vi "sample6(OPMode).vi"() -> ()   [LabVIEW 2011]
uses:
  <vilib>/Platform/TimedLoop/XDataNode/timing_clust.ctl
  <vilib>/Platform/TimedLoop/XDataNode/nitl_modes.ctl
  <vilib>/Platform/TimedLoop/XDataNode/wakeup.ctl
  <vilib>/Platform/TimedLoop/XDataNode/XDataNode.xnode
  <vilib>/Platform/TimedLoop/XDataNode/XDNodeRunTimeDep.lvlib
  user32.dll
panel:
  in  "Mode":u8(slide) scale=0.0..3.0
  out "change mode":bool
  out "Chart":cluster{"MovingSpeed":i16, "Present Speed":i16}(graph)
  out "Present Value":i16
  out "STOP2":bool
  in  "ID":u8=1 max=253
  in  "Baudrate":u32=1000000
  in  "COM":refnum<visa-resource-name> caption="COMポート"
  in  "STOP":bool
  in  "Value":i16(knob) scale=0.0..4095.0
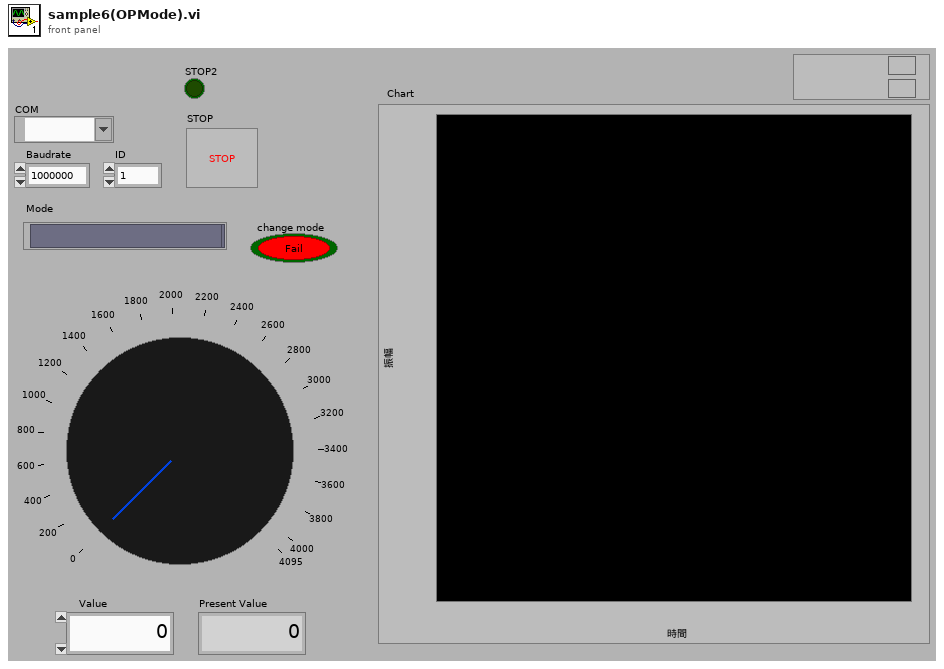
[diagram p1: front panel]
types:
  T1 = typedef "XDNodeRunTimeDep.lvlib/timing_clust.ctl" = cluster{"Expected End [f-1]":u64, "Actual End [f-1]":u64, "Finished Late? [f-1]":bool, "Expected End [i-1]":u64, "Actual End [i-1]":u64, "Finished Late? [i-1]":bool, "Expected Start [i]":u64, "Actual Start [i]":u64, "Expected Start [f]":u64, "Actual Start [f]":u64, "Source Name":string, "Structure Name":string, "Period":i64, "Deadline":i64, "Offset":i64, "Start":i64, "Priority":i32, "Timeout":i32, "Mode":T2, "Wakeup Reason":T3, "Error":errorcluster, "Source Type":string, "Secondary Source Type":string, "Global End Time":u64, "Global Start Time":u64, "Frame Duration":u64, "Iteration Duration":u64, "Assigned CPU":i32, "I/O Scan Engine Mode":u32}
  T2 = typedef "XDNodeRunTimeDep.lvlib/nitl_modes.ctl" = enum32{"No Change", "Process missed periods, maintain original phase", "Discard missed periods, maintain original phase", "Process missed periods, ignore original phase", "Discard missed periods, ignore original phase"}
  T3 = typedef "XDNodeRunTimeDep.lvlib/wakeup.ctl" = enum32{"Normal", "Aborted", "Asynchronous wakeup", "Timing source error", "Timed loop error", "Timeout"}
  T4 = enum16{"Joint", "Wheel", "Multi Turn", "unknown"}
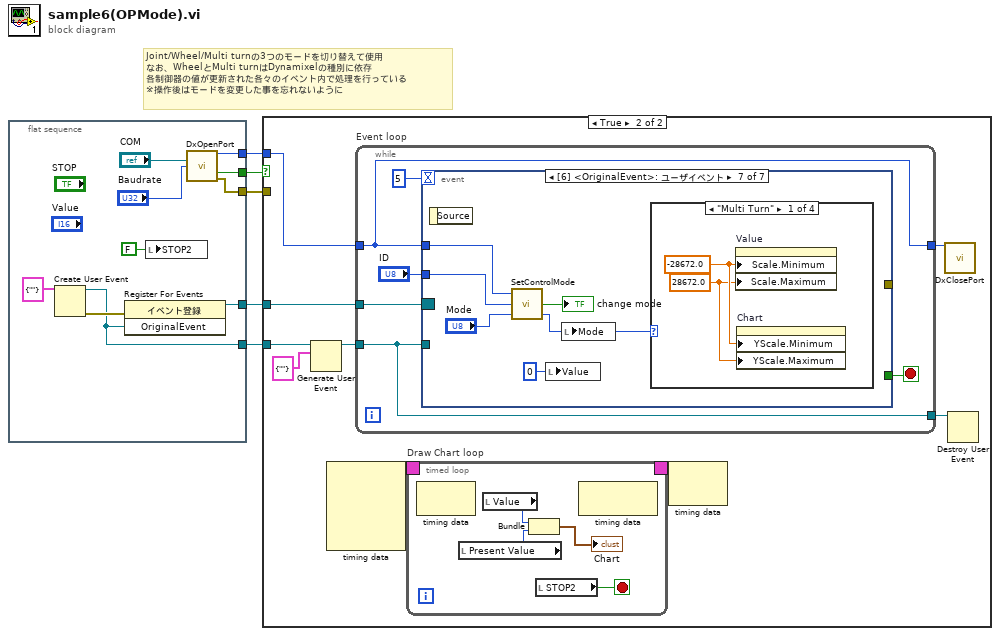
[diagram p0: block diagram]
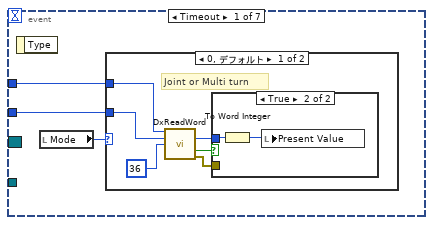
[diagram p3: hidden frame]
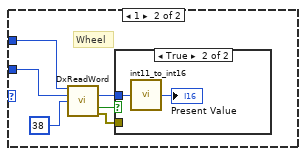
[diagram p5: hidden frame]
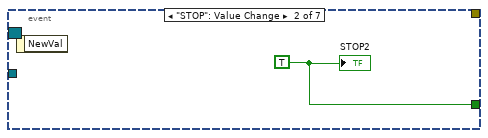
[diagram p7: hidden frame]
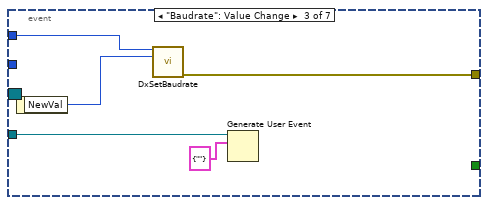
[diagram p8: hidden frame]
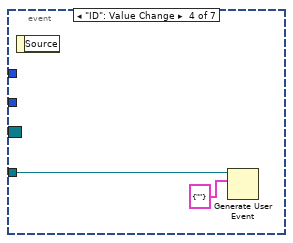
[diagram p9: hidden frame]
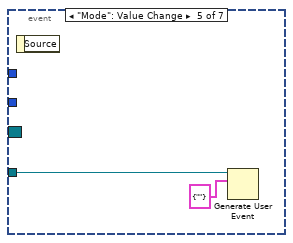
[diagram p10: hidden frame]
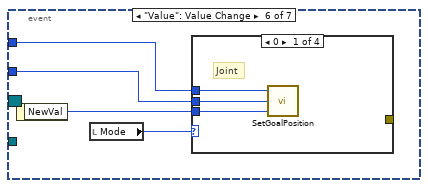
[diagram p11: hidden frame]
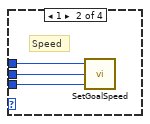
[diagram p12: hidden frame]
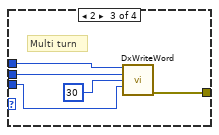
[diagram p13: hidden frame]
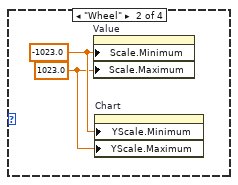
[diagram p15: hidden frame]
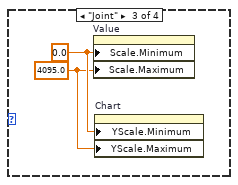
[diagram p16: hidden frame]
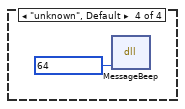
[diagram p17: hidden frame]
diagram:
  # "Joint/Wheel/Multi turnの3つのモードを切り替えて使用\nなお、WheelとMulti turnはDynamixelの種別に依存\n各制御器の値が更新された各々のイベント内で処理を行っている\n※操作後はモードを変更した事を忘れないように"
  n1 = flat-sequence {
    tunnel: [w13] -> w5
    tunnel: [w12] -> w4
    tunnel: [w11] -> w3
    tunnel: [w7] -> w2
    tunnel: [w6] -> w1
    frame #0 {
      n2 = Create User Event(user event datatype=cluster{"string":string} {"string"=""} ("OriginalEvent")) -> (user event=w6:refnum<user-event>, error out=w9:errorcluster)  [unwired: 1 in]
      n3 = register-events(error in=w9, w6) -> (reference out=w7:refnum<event-registration>)  [unwired: 1 in, 1 out]
      n4 = local write "STOP2"(FALSE ("STOP2")) -> ()
      n5 = call "DxOpenPort.vi"("port"="COM", "baudrate"="Baudrate") -> ("dvid"=w13:u32, "成功"=w12:bool, "エラー出力"=w11:errorcluster)  [unwired: 11 in]
    }
  }
  n6 = case shown="TRUE" w4 {
    tunnel: w5 -> [_ w22]
    tunnel: w3 -> [_ _]
    tunnel: w2 -> [_ w20]
    tunnel: w1 -> [_ w18]
    frame False {
    }
    frame True {
      n7 = Generate User Event(user event=w18, event data cluster=cluster{"string":string} {"string"=""} ("イベントデータ")) -> (user event out=w17:refnum<user-event>)  [unwired: 1 in, 1 out]
      n8 = node-c288() -> (w24:T1)  [unwired: 4 in]
      n9 = while "Event loop" {
        tunnel: w22 -> [w25]
        tunnel: [w25] -> w21
        tunnel: w20 -> [w27]
        tunnel: w17 -> [w26]
        tunnel: [w26] -> w16
        stop <- w30 stop-if-true
        n10 = event shown="[6] <OriginalEvent>: ユーザイベント" {
          selector: w27 -> [_ _ _ _ _ _ _]
          dyn-events: _ -> [_ _ _ _ _ _ _]
          timeout: 5 -> [_ _ _ _ _ _ _]
          tunnel: w25 -> [w33 _ w55 _ _ w62 w80]
          tunnel: [_ w50 _ _ _ _ _] -> w30
          tunnel: "ID" -> [w32 _ _ _ _ w60 w75]
          tunnel: w26 -> [_ _ w52 w56 w58 _ _]
          tunnel: [_ _ w51 _ _ _ _] -> _
          event Timeout {
            n11 = event-data() -> ()  [unwired: 1 in, 1 out]
            n12 = local read "Mode"() -> (w31:u8)
            n13 = case shown="0, デフォルト" w31 {
              tunnel: w33 -> [w35 w43]
              tunnel: w32 -> [w34 w42]
              frame 0, Default {
                # "Joint or Multi turn"
                n14 = call "DxReadWord.vi"("dvid in"=w35, "id"=w34, "address"=u16 36) -> ("data out"=w37:u16, "成功"=w38:bool, "エラー出力"=w39:errorcluster)  [unwired: 9 in, 1 out]
                n15 = case shown="TRUE" w38 {
                  tunnel: w37 -> [_ w41]
                  tunnel: w39 -> [_ _]
                  frame False {
                  }
                  frame True {
                    n16 = To Word Integer(number=w41) -> (16bit integer=w40:i16)
                    n17 = local write "Present Value"(w40) -> ()
                  }
                }
              }
              frame 1 {
                # "Wheel"
                n18 = call "DxReadWord.vi"("dvid in"=w43, "id"=w42, "address"=u16 38) -> ("data out"=w45:u16, "成功"=w46:bool, "エラー出力"=w47:errorcluster)  [unwired: 9 in, 1 out]
                n19 = case shown="TRUE" w46 {
                  tunnel: w45 -> [_ w48]
                  tunnel: w47 -> [_ _]
                  frame False {
                  }
                  frame True {
                    n20 = call "int11_to_int16.vi"("int11"=w48) -> ("int16"=→"Present Value":i16)
                  }
                }
              }
            }
          }
          event "STOP": Value Change {
            w50 = TRUE ("STOP2")
            n21 = event-data() -> ()  [unwired: 1 in, 1 out]
            "STOP2" <- w50
          }
          event "Baudrate": Value Change {
            n22 = event-data() -> ("NewVal"=w54:u32)  [unwired: 1 in]
            n23 = call "DxSetBaudrate.vi"("dvid in"=w55, "Baudrate"=w54) -> ("エラー出力"=w51:errorcluster)  [unwired: 11 in, 2 out]
            n24 = Generate User Event(user event=w52, event data cluster=cluster{"string":string} {"string"=""} ("イベントデータ")) -> ()  [unwired: 1 in, 2 out]
          }
          event "ID": Value Change {
            n25 = event-data() -> ()  [unwired: 1 in, 1 out]
            n26 = Generate User Event(user event=w56, event data cluster=cluster{"string":string} {"string"=""} ("イベントデータ")) -> ()  [unwired: 1 in, 2 out]
          }
          event "Mode": Value Change {
            n27 = event-data() -> ()  [unwired: 1 in, 1 out]
            n28 = Generate User Event(user event=w58, event data cluster=cluster{"string":string} {"string"=""} ("イベントデータ")) -> ()  [unwired: 1 in, 2 out]
          }
          event "Value": Value Change {
            n29 = event-data() -> ("NewVal"=w63:i16)  [unwired: 1 in]
            n30 = local read "Mode"() -> (w61:u8)
            n31 = case shown="0" w61 {
              tunnel: w63 -> [w64 w69 w71 _]
              tunnel: w60 -> [w65 w68 w72 _]
              tunnel: w62 -> [w66 w67 w73 _]
              tunnel: [_ _ w70 _] -> _
              frame 0 {
                # "Joint"
                n32 = call "SetGoalPosition.vi"("goal position"=w64, "Target ID"=w65, "dvid in"=w66) -> ()  [unwired: 1 in, 2 out]
              }
              frame 1 {
                # "Speed"
                n33 = call "SetGoalSpeed.vi"("goal speed"=w69, "Target ID"=w68, "dvid in"=w67) -> ()  [unwired: 1 in, 2 out]
              }
              frame 2 {
                # "Multi turn"
                n34 = call "DxWriteWord.vi"("dvid in"=w73, "id"=w72, "address"=u16 30, "data in"=w71) -> ("エラー出力"=w70:errorcluster)  [unwired: 9 in, 2 out]
              }
              frame 3, Default {
              }
            }
          }
          event User Event {
            n35 = event-data() -> ()  [unwired: 1 in, 1 out]
            n36 = call "SetControlMode.vi"("Mode"="Mode", "Target ID"=w75, "dvid in"=w80) -> ("Mode out"=w78:T4, "ok"=→"change mode":bool)  [unwired: 1 out]
            n37 = local write "Value"(i16 0 ("Value")) -> ()
            n38 = local write "Mode"(w78) -> ()
            n39 = case shown="\"Multi Turn\"" w78 {
              frame "Multi Turn" {
                w81 = 28672.0 ("スケール.範囲:最大値")
                w82 = -28672.0 ("スケール.範囲:最小値")
                n40 = property on="Value" class="Knob （指定）"("Scale.Minimum"=w82, "Scale.Maximum"=w81) -> ()  [unwired: 2 in, 2 out]
                n41 = property on="Chart" class="WFChart （指定）"("YScale.Minimum"=w82, "YScale.Maximum"=w81) -> ()  [unwired: 2 in, 2 out]
              }
              frame "Wheel" {
                w83 = 1023.0 ("スケール.範囲:最大値")
                w84 = -1023.0 ("スケール.範囲:最小値")
                n42 = property on="Value" class="Knob （指定）"("Scale.Minimum"=w84, "Scale.Maximum"=w83) -> ()  [unwired: 2 in, 2 out]
                n43 = property on="Chart" class="WFChart （指定）"("YScale.Minimum"=w84, "YScale.Maximum"=w83) -> ()  [unwired: 2 in, 2 out]
              }
              frame "Joint" {
                w85 = 4095.0 ("スケール.範囲:最大値")
                w86 = 0.0 ("スケール.範囲:最小値")
                n44 = property on="Value" class="Knob （指定）"("Scale.Minimum"=w86, "Scale.Maximum"=w85) -> ()  [unwired: 2 in, 2 out]
                n45 = property on="Chart" class="WFChart （指定）"("YScale.Minimum"=w86, "YScale.Maximum"=w85) -> ()  [unwired: 2 in, 2 out]
              }
              frame "unknown", Default {
                n46 = dll-call lib="user32.dll" fn="MessageBeep"("uType"=u32 64) -> ()  [unwired: 5 in, 2 out]
              }
            }
          }
        }
      }
      n47 = timed-loop "Draw Chart loop" {
        timing: w24 -> [_]
        timing-out: [_] -> w23
        stop <- w91 stop-if-true
        n48 = node-c288() -> ()  [unwired: 1 in, 1 out]
        n49 = local read "Present Value"() -> (w89:i16)
        n50 = local read "Value"() -> (w90:i16)
        n51 = Bundle("Value"=w90, "Present Value"=w89) -> (→"Chart":cluster{"Value":i16, "Present Value":i16})  [unwired: 1 in]
        n52 = local read "STOP2"() -> (w91:bool)
        n53 = node-c288() -> ()  [unwired: 1 in, 1 out]
      }
      n54 = node-c288(w23) -> ()  [unwired: 1 out]
      n55 = call "DxClosePort.vi"("dvid"=w21) -> ()  [unwired: 13 in, 2 out]
      n56 = Destroy User Event(user event=w16) -> ()  [unwired: 1 in, 1 out]
    }
  }
